vi "On-the-fly averages value update.vi"(1 "Logging queue element in":T1={"Imaging Protocol"=enum."Live Imaging", "Number of Trials"=0, "Frame Size"=512, "# Averaged frames"=0, "Dwell time (us)"=0.0, "Index of Z-plane"=0, "Timelapse?"=FALSE, "Logging process is active"=FALSE, "Speed logging enabled"=FALSE, "tdms file ref"=refnum, "path"=path "", "Trial Number"=0, "Expected # points acquired"=FALSE, "Manually stopped"=FALSE, "Ch0 data"=[], "Ch1 data"=[], "Last trial"=FALSE, "Points acquired"={"Ch0 last trial"=0, "Ch1 last trial"=0, "All trials"=0}} {"Frame Size" items=["100X100"=100, "128X128"=128, "200X200"=200, "256X256"=256, "512X512"=512, "1024x1024"=1024, "2048x2048"=2048]; "Dwell time (us)" format="%#.6g"}) -> (0 "Logging queue element":T1={"Imaging Protocol"=enum."Live Imaging", "Number of Trials"=0, "Frame Size"=512, "# Averaged frames"=0, "Dwell time (us)"=0.0, "Index of Z-plane"=0, "Timelapse?"=FALSE, "Logging process is active"=FALSE, "Speed logging enabled"=FALSE, "tdms file ref"=refnum, "path"=path "", "Trial Number"=0, "Expected # points acquired"=FALSE, "Manually stopped"=FALSE, "Ch0 data"=[], "Ch1 data"=[], "Last trial"=FALSE, "Points acquired"={"Ch0 last trial"=0, "Ch1 last trial"=0, "All trials"=0}} {"Frame Size" items=["100X100"=100, "128X128"=128, "200X200"=200, "256X256"=256, "512X512"=512, "1024x1024"=1024, "2048x2048"=2048]; "Dwell time (us)" format="%#.6g"})   [LabVIEW 2013]
uses:
  Typedefs/Logging queue element.ctl
  Typedefs/Imaging Protocols enum.ctl
  Typedefs/Frame Size.ctl
  Typedefs/Acquired points count.ctl
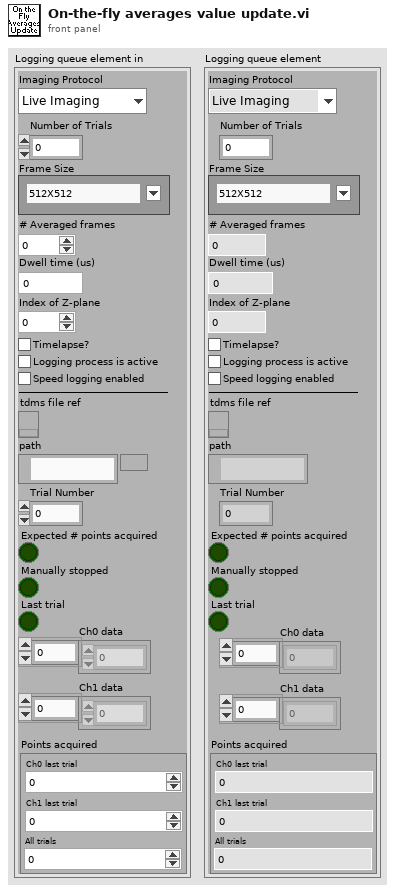
[diagram p1: front panel]
types:
  T1 = typedef "Logging queue element.ctl" = cluster{"Imaging Protocol":T2, "Number of Trials":u16, "Frame Size":T3, "# Averaged frames":u16, "Dwell time (us)":dbl, "Index of Z-plane":i32, "Timelapse?":bool, "Logging process is active":bool, "Speed logging enabled":bool, "tdms file ref":refnum<k34>, "path":path, "Trial Number":i32, "Expected # points acquired":bool, "Manually stopped":bool, "Ch0 data":u32[], "Ch1 data":u32[], "Last trial":bool, "Points acquired":T4}
  T2 = typedef "Imaging Protocols enum.ctl" = enum16{"AOL Z-Stack", "Motor Z Stack", "Functional Acquisition", "Single Plane Acquisition", "Volume Acquisition", "Live Imaging", "Live Plane Imaging", "Live Volume Imaging"}
  T3 = typedef "Frame Size.ctl" = u16
  T4 = typedef "Acquired points count.ctl" = cluster{"Ch0 last trial":u64, "Ch1 last trial":u64, "All trials":u64}
  T5 = typedef "AOL_Globals.ctl" = cluster{"Imaging Protocol":T2, "Number of POI":u16, "Number of Miniscans":u16, "Number of Trials":u16, "Number of Cycles ":u64, "# Averaged Frames":u16, "Laser power (%)":u8, "Pockels":dbl, "Acquisition Length (sec)":dbl, "Fill time (us)":dbl, "POI Dwell time (us)":dbl, "Miniscan Dwell time per pixel (us)":dbl, "PMT 1":dbl, "PMT 2":dbl, "Back Apperture":dbl, "Frame Size":T3, "Center Frequency":dbl, "Field of View":dbl, "DwellTime (us)":dbl, "Wavelength (nm)":dbl, "Zoom":dbl, "AOL Z":dbl, "AOL Mode":T6, "GridXY":dbl, "GridZ":dbl, "TriggerPeriod (sec)":dbl, "Number of Pixels in Miniscan":u16, "Experiment folder path":path, "X centre":dbl, "Y centre":dbl, "Angle (degrees)":dbl, "Plane Mode":T7, "Threshold":u16[], "Regenerate Chirps":bool, "Rectangle ROI length (pixels)":u16, "Rectangle ROI height (pixels)":u16, "AOD fill":u16, "Samples Wait after Trigger":u16, "StartUp Delay":i32, "Slip Cycle":u32, "Add Cycle":bool}
  T6 = typedef "AOL modes.ctl" = enum16{"Raster", "Structural", "Pointing", "Mini Scan", "Alignment"}
  T7 = typedef "Plane Mode.ctl" = u16
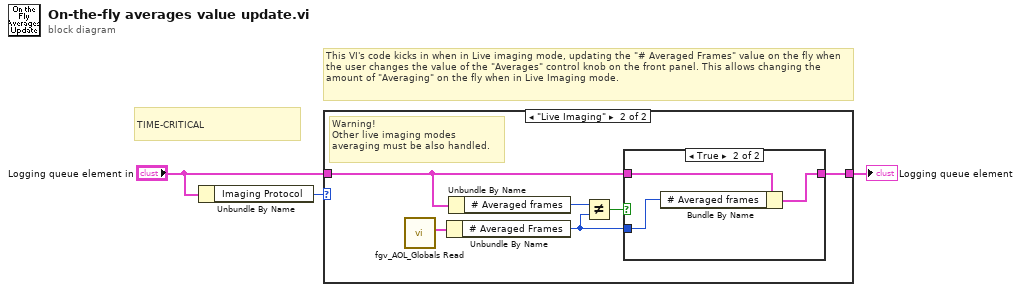
[diagram p0: block diagram]
diagram:
  # "TIME-CRITICAL"
  # "This VI's code kicks in when in Live imaging mode, updating the \"# Averaged Frames\" value on the fly when the user changes the value of the \"Averages\" control knob on the front panel. This allows changing the amount of \"Averaging\" on the fly when in Live Imaging mode."
  n1 = Unbundle By Name("Logging queue element in") -> ("Imaging Protocol"=w2:T2)
  n2 = case shown="\"Live Imaging\"" w2 {
    tunnel: "Logging queue element in" -> [w4 w7]
    tunnel: [w4 w5] -> w1
    frame Default {
    }
    frame "Live Imaging" {
      # "Warning!\nOther live imaging modes\naveraging must be also handled."
      n3 = call "fgv_AOL_Globals Read.vi"() -> ("AOL_Globals"=w10:T5)  [unwired: 9 in, 2 out]
      n4 = Unbundle By Name(w10) -> ("# Averaged Frames"=w6:u16)
      n5 = Unbundle By Name(w7) -> ("# Averaged frames"=w9:u16)
      n6 = Not Equal?(x=w9, y=w6) -> (x != y?=w8:bool)
      n7 = case shown="True" w8 {
        tunnel: w7 -> [w11 w14]
        tunnel: w6 -> [_ w13]
        tunnel: [w11 w12] -> w5
        frame False {
        }
        frame True {
          n8 = Bundle By Name(cluster=w14, "# Averaged frames"=w13) -> (w12:T1)
        }
      }
    }
  }
  "Logging queue element" <- w1
